vi "POVToBoolean.vi"(10 "Input":i32) -> (2 "Output":T1)   [LabVIEW 2014]
doc: "Given the numeric input from a POV on a joystick, returns a cluster of named booleans that lets you probe the values you want.\n\nThe center value of the POV is MiddleCenter."
panel:
  in  "Cluster":T1
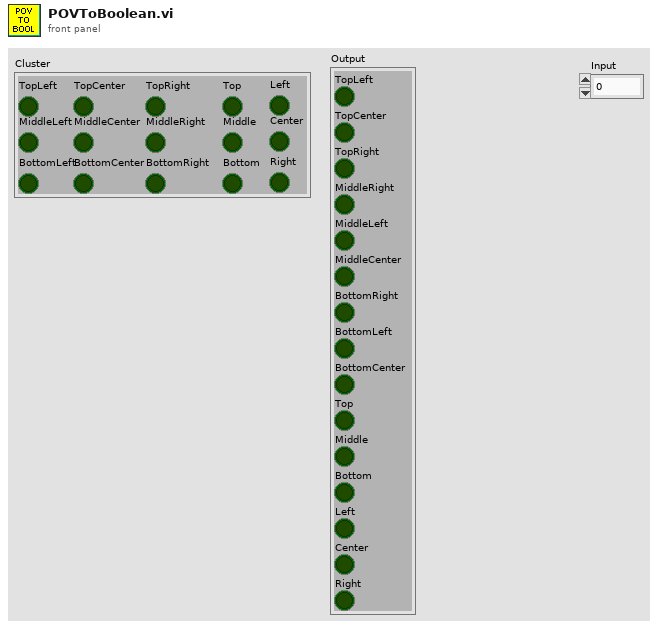
[diagram p1: front panel]
types:
  T1 = cluster{"TopLeft":bool, "TopCenter":bool, "TopRight":bool, "MiddleRight":bool, "MiddleLeft":bool, "MiddleCenter":bool, "BottomRight":bool, "BottomLeft":bool, "BottomCenter":bool, "Top":bool, "Middle":bool, "Bottom":bool, "Left":bool, "Center":bool, "Right":bool}
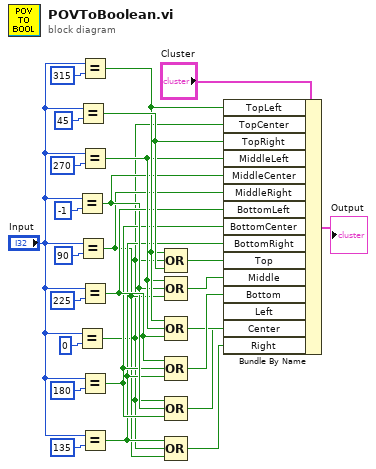
[diagram p0: block diagram]
diagram:
  n1 = Equal?(x="Input", y=i16 -1) -> (x = y?=w7:bool)
  n2 = Equal?(x="Input", y=i16 0) -> (x = y?=w2:bool)
  n3 = Equal?(x="Input", y=i16 45) -> (x = y?=w15:bool)
  n4 = Equal?(x="Input", y=i16 90) -> (x = y?=w3:bool)
  n5 = Equal?(x="Input", y=i16 315) -> (x = y?=w12:bool)
  n6 = Equal?(x="Input", y=i16 270) -> (x = y?=w11:bool)
  n7 = Equal?(x="Input", y=i16 225) -> (x = y?=w10:bool)
  n8 = Equal?(x="Input", y=i16 180) -> (x = y?=w6:bool)
  n9 = Equal?(x="Input", y=i16 135) -> (x = y?=w4:bool)
  n10 = Compound Arithmetic op=OR(w12, w2, w15) -> (w16:bool)
  n11 = Compound Arithmetic op=OR(w11, w7, w3) -> (w14:bool)
  n12 = Compound Arithmetic op=OR(w12, w11, w10) -> (w9:bool)
  n13 = Compound Arithmetic op=OR(w10, w6, w4) -> (w13:bool)
  n14 = Compound Arithmetic op=OR(w2, w7, w6) -> (w8:bool)
  n15 = Compound Arithmetic op=OR(w4, w2, w3) -> (w5:bool)
  n16 = Bundle By Name(cluster="Cluster", "TopLeft"=w12, "TopCenter"=w2, "TopRight"=w15, "MiddleLeft"=w11, "MiddleCenter"=w7, "MiddleRight"=w3, "BottomLeft"=w10, "BottomCenter"=w6, "BottomRight"=w4, "Top"=w16, "Middle"=w14, "Bottom"=w13, "Left"=w9, "Center"=w8, "Right"=w5) -> (→"Output":T1)
